vi "Evaluate Part 2.vi"() -> ()   [LabVIEW 2020]
uses:
  Schema Parser/Schema Parser.lvclass
  Number/Number.lvclass
  Symbol/Symbol.lvclass
panel:
  out "sum":i32=467835
  in  "String":string="467..114..\n...*......\n..35..633.\n......#...\n617*......\n.....+.58.\n..592.....\n......755.\n...$.*....\n.664.598.."
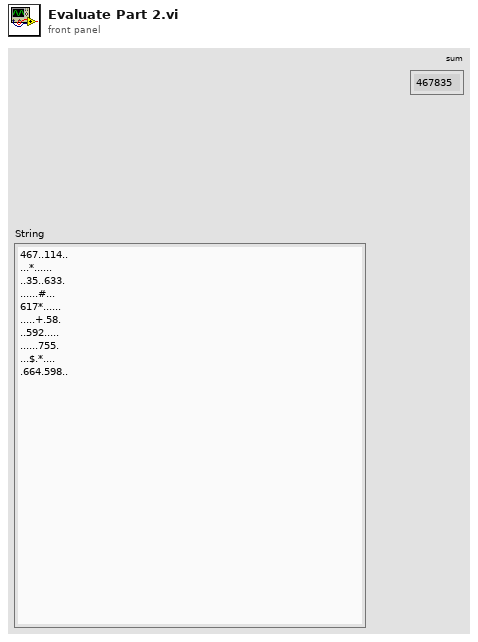
[diagram p1: front panel]
types:
  T1 = cluster{"Number":refnum<class "Number.lvclass">, "Number 2":refnum<class "Number.lvclass">}[]
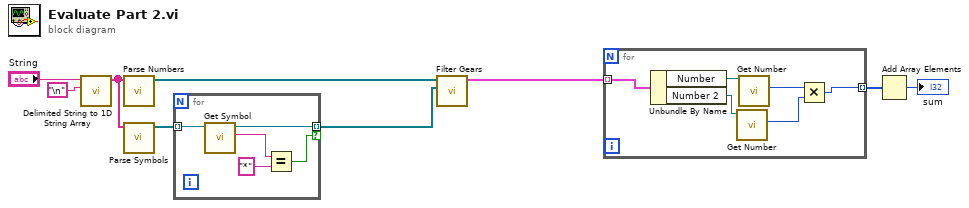
[diagram p0: block diagram]
diagram:
  n1 = call <vilib>:"Delimited String to 1D String Array.vi"("delimiter"="\n", "delimited string"="String") -> ("string array"=w7:string[])  [unwired: 9 in]
  n2 = call "Parse Numbers.vi"("string array"=w7) -> ("Array"=w6:refnum<class "Number.lvclass">[])  [unwired: 10 in]
  n3 = call "Parse Symbols.vi"("string array"=w7) -> ("Array"=w5:refnum<class "Symbol.lvclass">[])  [unwired: 10 in]
  n4 = for {
    tunnel: w5 -> [w14] mode=indexing
    tunnel: [w13] -> w1 mode=indexing if=w10
    n5 = call "Get Symbol.vi"("Symbol in"=w14) -> ("Symbol"=w12:string, "Symbol out"=w13:refnum<class "Symbol.lvclass">)  [unwired: 8 in, 1 out]
    n6 = Equal?(x=w12, y="*") -> (x = y?=w10:bool)
  }
  n7 = call "Filter Gears.vi"("Symbols"=w1, "Numbers"=w6) -> ("Gears"=w4:T1)  [unwired: 9 in]
  n8 = for {
    tunnel: w4 -> [w19] mode=indexing
    tunnel: [w16] -> w3 mode=indexing
    n9 = Unbundle By Name(w19) -> ("Number"=w18:refnum<class "Number.lvclass">, "Number 2"=w17:refnum<class "Number.lvclass">)
    n10 = call "Get Number.vi"("Number in"=w17) -> ("Number"=w15:i32)  [unwired: 8 in, 2 out]
    n11 = call "Get Number.vi"("Number in"=w18) -> ("Number"=w20:i32)  [unwired: 8 in, 2 out]
    n12 = Multiply(x=w20, y=w15) -> (x*y=w16:i32)
  }
  n13 = Add Array Elements(numeric array=w3) -> (sum=→"sum":i32)
